vi "Reset Contestant Lights.vi"(8 "error in (no error)":errorcluster, 11 "Controller in":refnum<class "Controller.lvclass">) -> (0 "error out":errorcluster, 3 "Controller out":refnum<class "Controller.lvclass">)   [LabVIEW 2021, in "Controller.lvlib" / "Controller.lvclass"]
uses:
  Controller.lvclass
  Controller.lvclass/Controller.ctl
  <vilib>/ActorFramework/Message Enqueuer/Message Enqueuer.lvclass/Message Enqueuer.ctl
  <vilib>/ActorFramework/Message Enqueuer/Enqueue.vi
  Contestant/Contestant Messages/Light to Nuetral Msg/Light to Nuetral Msg.lvclass
  C:/Program Files/National Instruments/LabVIEW 2024/vi.lib/ActorFramework/Message/Message.lvclass
  <vilib>/ActorFramework/Message Priority Queue/Priority Enqueue.vi
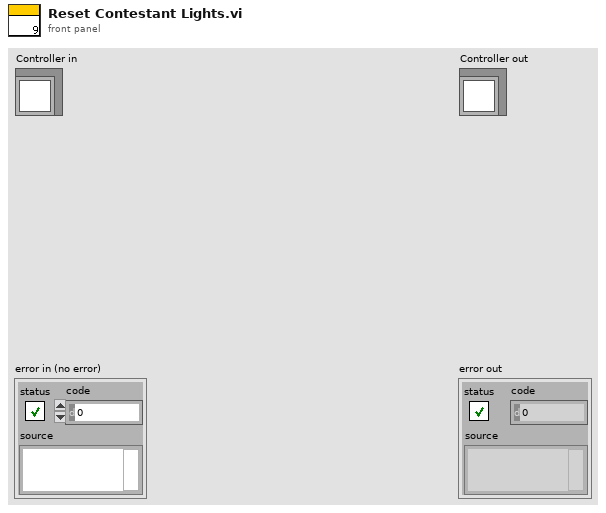
[diagram p1: front panel]
types:
  T1 = map{i32, refnum<class "Message Enqueuer.lvclass">}
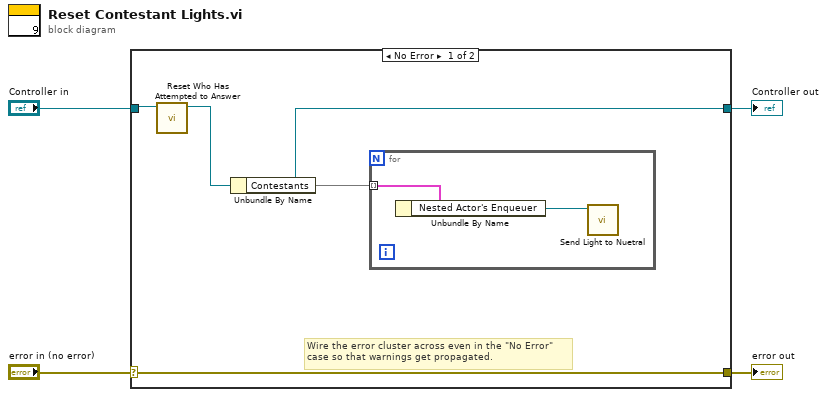
[diagram p0: block diagram]
diagram:
  n1 = case shown="No Error" "error in (no error)" {
    selector: "error in (no error)" -> [w8 w12]
    tunnel: [w8 w12] -> w3
    tunnel: [w5 w11] -> w1
    tunnel: "Controller in" -> [w6 w11]
    frame No Error {
      # "Wire the error cluster across even in the \"No Error\"\ncase so that warnings get propagated."
      n2 = call-dynamic "Reset Who Has Attempted to Answer.vi"("Controller in"=w6) -> ("Controller out"=w5:refnum<class "Controller.lvclass">)  [unwired: 9 in, 1 out]
      n3 = Unbundle By Name(w5) -> ("Contestants"=w7:T1)
      n4 = for {
        tunnel: w7 -> [w10] mode=indexing
        n5 = Unbundle By Name(w10) -> ("Nested Actor's Enqueuer"=w9:refnum<class "Message Enqueuer.lvclass">)
        n6 = call "Send Light to Nuetral.vi"("Message Enqueuer"=w9) -> ()  [unwired: 9 in, 2 out]
      }
    }
    frame Error {
    }
  }
  "error out" <- w3
  "Controller out" <- w1
